vi "Select_API_Commands.vi"(1 "Input Selection":i32[](array[numeric]), 2 "Input Sequence":cluster{string, string[], dbl[], dbl}[](array[cluster])) -> (0 "Output Selection":i32[](array[numeric]))   [LabVIEW 2011]
doc: "This VI examines the \"Input Selection\" (an array of indices in the input sequence), and if it finds any API commands with the same ID as a selected command, adds those API commands to the \"Output Selection\"."
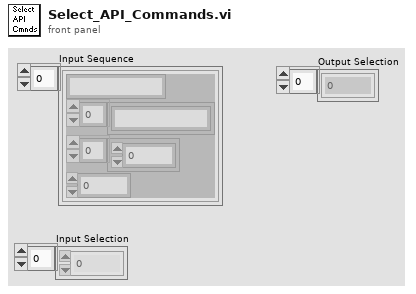
[diagram p1: front panel]
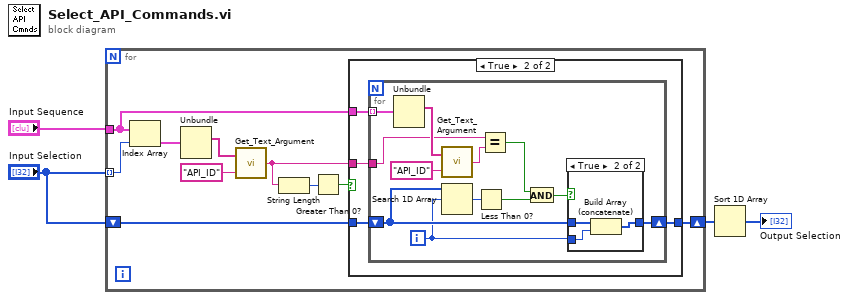
[diagram p0: block diagram]
diagram:
  n1 = for {
    tunnel: "Input Selection" -> [w7] mode=indexing
    tunnel: "Input Sequence" -> [w13]
    shift-right: [w6] -> w1
    shift-left: "Input Selection" -> [w5]
    n2 = Index Array(array=w13, index=w7) -> (element=w11:cluster{string, string[], dbl[], dbl})
    n3 = Unbundle(w11) -> (w12:string[])  [unwired: 3 out]
    n4 = call "Get_Text_Argument.vi"("Argument"="API_ID", "Argument List"=w12) -> ("Text"=w10:string)
    n5 = String Length(string=w10) -> (length=w8:i32)
    n6 = Greater Than 0?(x=w8) -> (x > 0?=w9:bool)
    n7 = case shown="True" w9 {
      tunnel: w13 -> [_ w19]
      tunnel: w5 -> [w15 w18]
      tunnel: w10 -> [_ w17]
      tunnel: [w15 w16] -> w6
      frame False {
      }
      frame True {
        n8 = for {
          tunnel: w19 -> [w31] mode=indexing
          shift-right: [w26] -> w16
          shift-left: w18 -> [w25]
          tunnel: w17 -> [w27]
          i -> [w24]
          n9 = Unbundle(w31) -> (w29:string[])  [unwired: 3 out]
          n10 = call "Get_Text_Argument.vi"("Argument"="API_ID", "Argument List"=w29) -> ("Text"=w28:string)
          n11 = Search 1D Array(1D array=w25, element=w24) -> (index of element=w23:i32)  [unwired: 1 in]
          n12 = Less Than 0?(x=w23) -> (x < 0?=w22:bool)
          n13 = Equal?(x=w27, y=w28) -> (x = y?=w21:bool)
          n14 = And(x=w21, y=w22) -> (x .and. y?=w20:bool)
          n15 = case shown="True" w20 {
            tunnel: w25 -> [w32 w35]
            tunnel: w24 -> [_ w34]
            tunnel: [w32 w33] -> w26
            frame False {
            }
            frame True {
              n16 = Build Array (concatenate)(w35, w34) -> (w33:i32[])
            }
          }
        }
      }
    }
  }
  n17 = Sort 1D Array(array=w1) -> (sorted array=→"Output Selection":i32[])
